vi "Koheras_Laser_switch.vi"(9 "Koheras Seed Laser":bool, 10 "Change-Detector in":bool, 11 "Modus in":i32) -> (0 "Answer Length Out":i32[](array[numeric]), 1 "Command Out":string[](array[string]), 3 "Modus Out":i32)   [LabVIEW 2009]
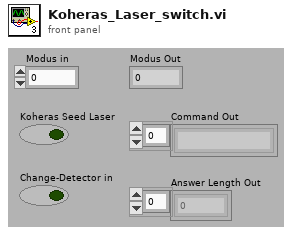
[diagram p1: front panel]
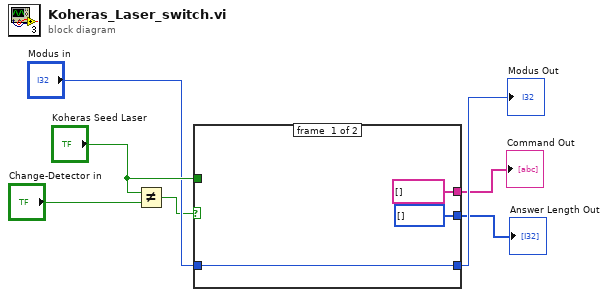
[diagram p0: block diagram]
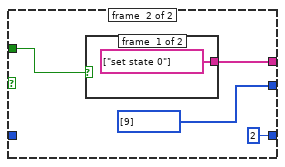
[diagram p2: hidden frame]
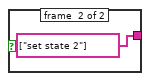
[diagram p3: hidden frame]
diagram:
  n1 = Not Equal?(x="Koheras Seed Laser", y="Change-Detector in") -> (x != y?=w4:bool)
  n2 = case shown="True" w4 {
    tunnel: "Koheras Seed Laser" -> [_ w14]
    tunnel: [string[] [] w13] -> w2
    tunnel: [i32[] [] i32[] [9]] -> w3
    tunnel: "Modus in" -> [w8 _]
    tunnel: [w8 2] -> w6
    frame #0 {
    }
    frame #1 {
      n3 = case shown="True" w14 {
        tunnel: [string[] ["set state 0"] string[] ["set state 2"]] -> w13
        frame #0 {
        }
        frame #1 {
        }
      }
    }
  }
  "Modus Out" <- w6
  "Answer Length Out" <- w3
  "Command Out" <- w2
